vi "RT Loop - Analyze Acceleration_V3.vi"(7 "testing":bool, 8 "error in (no error)":errorcluster, 9 "Acceleration RT FIFO In":T1, 10 "FPGA VI Reference Out 2":refnum<k20>, 11 "Message Queue":refnum<queue>) -> (1 "Acceleration RT FIFO Out":T1)   [LabVIEW 2017]
doc: "Read and analyze acceleration waveform data from FPGA via DMA FIFO. If the acceleration is over the limit, then send the acceleration waveform data to the Log Data Loop."
uses:
  UI Error Handlers/support/Message Queue/Message Cluster.ctl
  controls/Acceleration RT FIFO Reference.ctl
  data_sav.ctl
  Control 1.ctl
  Globals/Global - All RT Loop Stop.vi
  Globals/Global - Configuration Options.vi
  <vilib>/Utility/error.llb/Error Cluster From Error Code.vi
  <vilib>/rvi/errors/niLvFpgaAdjustHostInterfaceError.vi
  <vilib>/rvi/interface/nirviMethod/nirviMethod.xnode
  <vilib>/FPGAPlugInAG/Dynamic/niLvFpga_ReadFifo_Dynamic.vi
  <vilib>/rvi/errors/niLvFpgaMergeErrorWithErrorCode.vi
  UI Error Handlers/support/Logging/Logging.lvlib
  UI Error Handlers/support/Message Queue/Message Queue.lvlib
panel:
  out "error out 2":errorcluster
  out "error out":errorcluster
  out "x-y":u32
  out "G1 status":cluster{"G1 trigger":bool}
  out "G1 status.G1 trigger":bool
  out "sta":bool
  out "logical OR":bool
  in  "Data Rate (Hz)":dbl
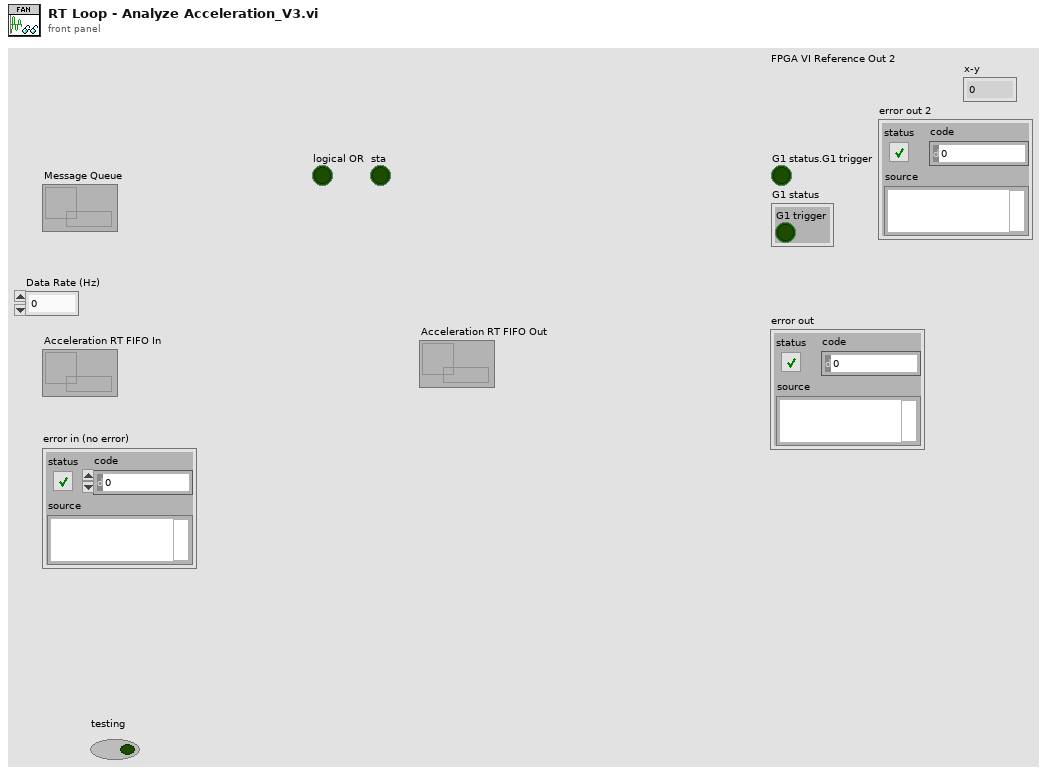
[diagram p1: front panel]
types:
  T1 = typedef "Acceleration RT FIFO Reference.ctl" = refnum<k33>
  T2 = typedef "data_sav.ctl" = cluster{"Log File out 2":refnum<k34>, "Array":T3[]}
  T3 = typedef "Control 1.ctl" = waveform(dbl)
  T4 = cluster{"Tool data":cluster{"Number of teeth":sgl}, "Cutting data":cluster{"rpm":sgl}, "Limits":cluster{"Magnitude threshold":sgl, "Tolerance":sgl}, "G1 status":cluster{"G1 trigger":bool}}
  T5 = cluster{"Log File out":refnum<k34>, waveform(dbl)[]}
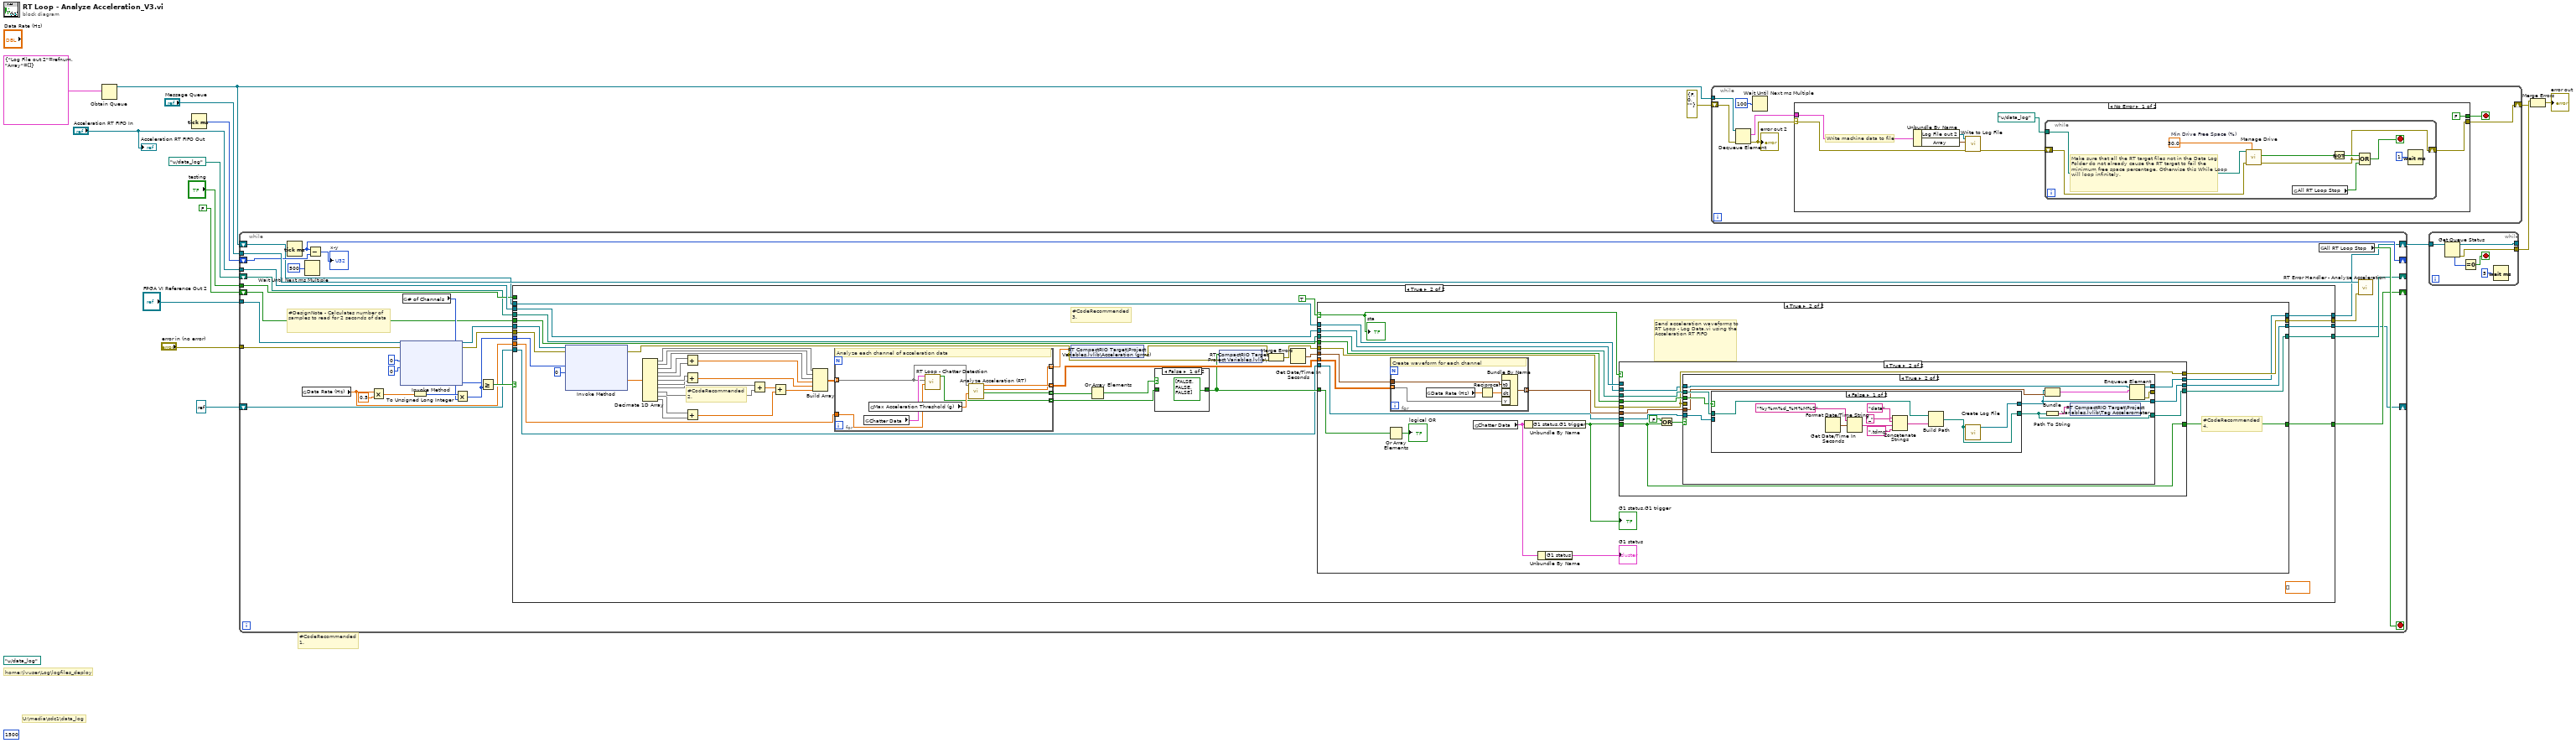
[diagram p0: block diagram]
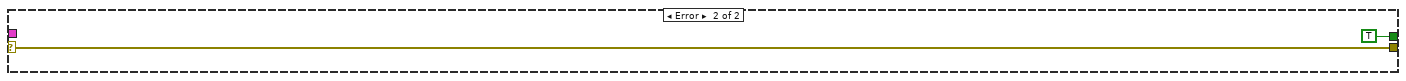
[diagram p2: hidden frame]
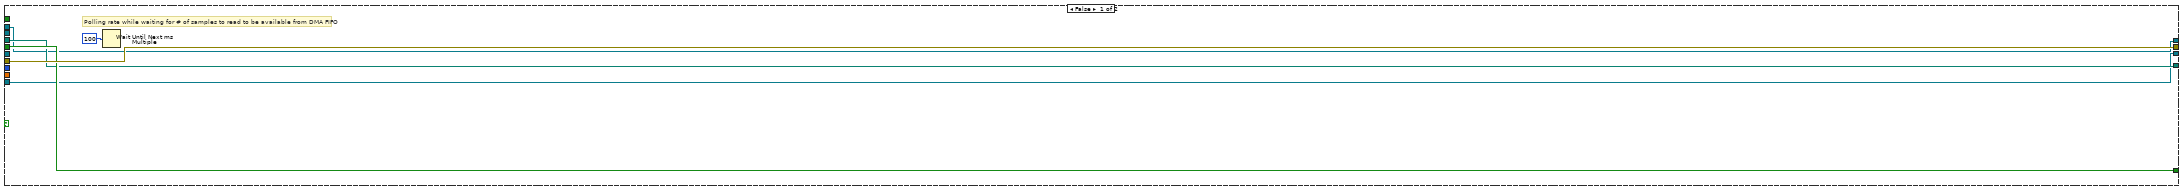
[diagram p3: hidden frame]
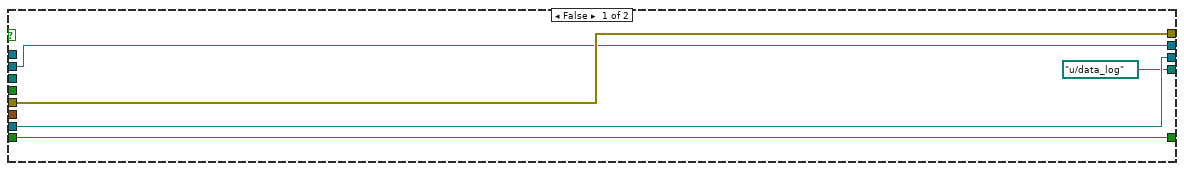
[diagram p6: hidden frame]
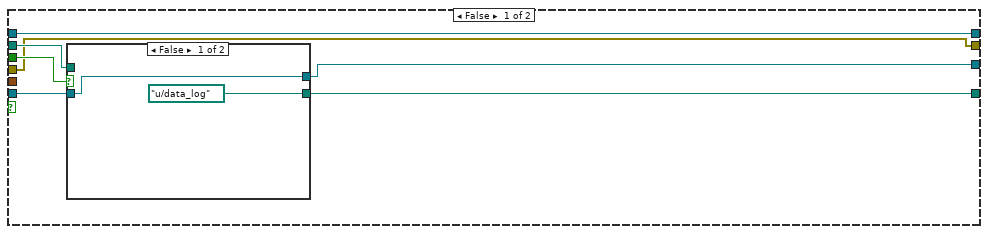
[diagram p7: hidden frame]
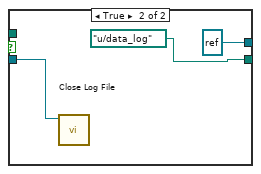
[diagram p8: hidden frame]
diagram:
  (unwired) 1500 ("max queue size (-1, unlimited)")
  (unwired) path "u:/data_log" ("AVI Path")
  # "U:\\media\\sdc1\\data_log"
  # "home:\\lvuser\\Log\\logfiles_deploy"
  # "#CodeRecommended\n1."
  n1 = Obtain Queue(element data type=T2 {"Log File out 2"=refnum, "Array"=[]}) -> (queue out=w5:refnum<queue>)  [unwired: 4 in, 2 out]
  n2 = Tick Count (ms)() -> (millisecond timer value=w9:u32)
  n3 = while {
    tunnel: "FPGA VI Reference Out 2" -> [w47]
    tunnel: "error in (no error)" -> [w46]
    tunnel: "Message Queue" -> [w39]
    tunnel: "Acceleration RT FIFO In" -> [w37]
    tunnel: "testing" -> [w29]
    shift-right: [w26] -> _
    shift-left: path "u:/data_log" ("AVI Path") -> [w25]
    shift-right: [w28] -> _
    shift-left: FALSE -> [w27]
    shift-right: [w24] -> _
    shift-left: refnum<k34> refnum ("Log File out") -> [w23]
    shift-right: [w21] -> _
    shift-left: w9 -> [w22]
    shift-right: [w18] -> w1
    shift-left: w5 -> [w19]
    stop <- w40 stop-if-true
    # "#DesignNote - Calculates number of samples to read for 2 seconds of data"
    n4 = Tick Count (ms)() -> (millisecond timer value=w21:u32)
    n5 = global read "Global - Configuration Options.vi" "Data Rate (Hz)"() -> (w31:dbl)
    n6 = Wait Until Next ms Multiple(millisecond multiple=u32 500) -> ()  [unwired: 1 out]
    n7 = Subtract(x=w21, y=w22) -> (x-y=→"x-y":u32)
    n8 = Multiply(x=w31, y=0.5) -> (x*y=w35:dbl)
    n9 = xnode "Invoke Method"("FPGA VI Reference In"=w47, "error in"=w46, "Number of Elements"=u32 0, "Timeout (ms)"=0) -> ("FPGA VI Reference Out"=w43:refnum<k20>, "error out"=w42:errorcluster, "Elements Remaining"=w30:u32)  [unwired: 1 out]
    n10 = global read "Global - Configuration Options.vi" "# of Channels"() -> (w32:u32)
    n11 = To Unsigned Long Integer(number=w35) -> (unsigned 32bit integer=w34:u32)
    n12 = Multiply(x=w34, y=w32) -> (x*y=w33:u32)
    n13 = Greater Or Equal?(x=w30, y=w33) -> (x >= y?=w41:bool)
    n14 = case shown="True" w41 {
      tunnel: w43 -> [_ w98]
      tunnel: w42 -> [w53 w97]
      tunnel: [w53 w93] -> w38
      tunnel: w33 -> [_ w96]
      tunnel: w37 -> [_ w91]
      tunnel: w31 -> [_ w88]
      tunnel: w29 -> [_ _]
      tunnel: [w51 w80] -> w28
      tunnel: w27 -> [w51 w79]
      tunnel: [w50 w78] -> w26
      tunnel: w25 -> [w50 w77]
      tunnel: [w49 w76] -> w24
      tunnel: w23 -> [w49 w75]
      tunnel: w19 -> [w48 w56]
      tunnel: [w48 w55] -> w18
      frame False {
        # "Polling rate while waiting for # of samples to read to be available from DMA FIFO"
        n15 = Wait Until Next ms Multiple(millisecond multiple=u32 100) -> ()  [unwired: 1 out]
      }
      frame True {
        (unwired) dbl[] []
        # "#CodeRecommended\n3."
        # "#CodeRecommended\n2."
        n16 = xnode "Invoke Method"("FPGA VI Reference In"=w98, "error in"=w97, "Number of Elements"=w96, "Timeout (ms)"=0) -> ("error out"=w87:errorcluster, "Data"=w90:sgl[])  [unwired: 2 out]
        n17 = Decimate 1D Array(w90) -> (w72:sgl[], w71:sgl[], w70:sgl[], w69:sgl[], w68:sgl[], w66:sgl[], w65:sgl[], w64:sgl[], w63:sgl[], w62:sgl[], w61:sgl[])
        n18 = Add(x=w69, y=w68) -> (x+y=w67:sgl[])
        n19 = Add(x=w66, y=w65) -> (x+y=w57:sgl[])
        n20 = Add(x=w62, y=w61) -> (x+y=w59:sgl[])
        n21 = Add(x=w64, y=w63) -> (x+y=w60:sgl[])
        n22 = Add(x=w60, y=w59) -> (x+y=w58:sgl[])
        n23 = Build Array(w72, w71, w70, w67, w57, w58) -> (w73:sgl[][])
        n24 = for {
          tunnel: [w108] -> w92 mode=indexing
          tunnel: [w107] -> w89 mode=indexing
          tunnel: [w106] -> w54 mode=indexing
          tunnel: w88 -> [w104]
          tunnel: [w103] -> w82 mode=indexing
          tunnel: w73 -> [w101] mode=indexing
          # "Analyze each channel of acceleration data"
          n25 = global read "Global - Configuration Options.vi" "Chatter Data"() -> (w102:T4)
          n26 = global read "Global - Configuration Options.vi" "Max Acceleration Threshold (g)"() -> (w105:sgl)
          n27 = call "RT Loop - Chatter Detection.vi"("Data Rate (Hz)"=w104, "Acceleration Waveform (SGL)"=w101, "Chatter Data"=w102) -> ("Chatter?"=w103:bool)  [unwired: 8 in]
          n28 = call "Analyze Acceleration (RT).vi"("Max Instantaneous Acceleration (g)"=w105, "Acceleration Waveform (SGL)"=w101) -> ("Over Limit?"=w108:bool, "Acceleration (grms)"=w106:dbl, "Acceleration Waveform (DBL)"=w107:dbl[])  [unwired: 7 in]
        }
        n29 = shared-variable "RT CompactRIO Target\\Project Variables.lvlib\\Acceleration (grms)"(w54, error in=w87) -> (error out=w85:errorcluster)
        n30 = Or Array Elements(Boolean array=w92) -> (logical OR=w83:bool)
        n31 = case shown="False" w83 {
          tunnel: w82 -> [_ w100]
          tunnel: [bool[] [FALSE, FALSE, FALSE] ("Chatter?") w100] -> w81
          frame False {
          }
          frame True {
          }
        }
        n32 = shared-variable "RT CompactRIO Target\\Project Variables.lvlib\\Chatter?"(w81, error in=w87) -> (error out=w86:errorcluster)
        n33 = Merge Errors(w85, w86) -> (w84:errorcluster)
        n34 = Get Date/Time In Seconds() -> (seconds since 1Jan1904=w94:timestamp)
        n35 = case shown="True" TRUE {
          selector: TRUE -> [_ w114]
          tunnel: w94 -> [_ w133]
          tunnel: w84 -> [w113 w132]
          tunnel: [w113 w117] -> w93
          tunnel: w91 -> [_ w130]
          tunnel: w89 -> [_ w129]
          tunnel: w81 -> [_ w127]
          tunnel: [w112 w124] -> w80
          tunnel: w79 -> [w112 w123]
          tunnel: [w111 w122] -> w78
          tunnel: w77 -> [w111 w118]
          tunnel: [w110 w121] -> w76
          tunnel: w75 -> [w110 w120]
          tunnel: w56 -> [w109 w116]
          tunnel: [w109 w115] -> w55
          frame False {
          }
          frame True {
            # "#CodeRecommended\n4."
            # "Send acceleration waveforms to RT Loop - Log Data.vi using the Acceleration RT FIFO"
            n36 = Or Array Elements(Boolean array=w127) -> (logical OR=→"logical OR":bool)
            n37 = for {
              tunnel: w129 -> [w190] mode=indexing
              tunnel: w133 -> [w189]
              tunnel: [w187] -> w131 mode=indexing
              # "Create waveform for each channel"
              n38 = global read "Global - Configuration Options.vi" "Data Rate (Hz)"() -> (w186:dbl)
              n39 = Reciprocal(x=w186) -> (1/x=w188:dbl)
              n40 = Bundle By Name("t0"=w189, "dt"=w188, "Y"=w190) -> (w187:waveform(dbl))  [unwired: 1 in]
            }
            n41 = global read "Global - Configuration Options.vi" "Chatter Data"() -> (w126:T4)
            n42 = Unbundle By Name(w126) -> ("G1 status.G1 trigger"=w119:bool)
            "G1 status.G1 trigger" <- w119
            n43 = Unbundle By Name(w126) -> ("G1 status"=→"G1 status":cluster{"G1 trigger":bool})
            n44 = case shown="True" w114 {
              tunnel: w132 -> [w138 w141]
              tunnel: w131 -> [_ w142]
              tunnel: w130 -> [_ _]
              tunnel: w119 -> [w136 w148]
              tunnel: [w136 w148] -> w124
              tunnel: w123 -> [_ w147]
              tunnel: [path "u:/data_log" ("AVI Path") w146] -> w122
              tunnel: w118 -> [_ w145]
              tunnel: [w137 w144] -> w121
              tunnel: w120 -> [w137 w143]
              tunnel: [w138 w141] -> w117
              tunnel: w116 -> [w134 w139]
              tunnel: [w134 w140] -> w115
              frame False {
              }
              frame True {
                n45 = Or(x=FALSE, y=w148) -> (x .or. y?=w150:bool)
                n46 = case shown="True" w150 {
                  tunnel: w145 -> [w154 w173]
                  tunnel: [w157 w170] -> w146
                  tunnel: w147 -> [w155 w172]
                  tunnel: w143 -> [w156 w164]
                  tunnel: w142 -> [_ w166]
                  tunnel: [w153 w163] -> w144
                  tunnel: w141 -> [w152 _]
                  tunnel: [w152 w169] -> _
                  tunnel: w139 -> [w151 w165]
                  tunnel: [w151 w168] -> w140
                  frame False {
                    n47 = case shown="False" w155 {
                      tunnel: [path "u:/data_log" ("AVI Path") path "u:/data_log" ("AVI Path")] -> w157
                      tunnel: w156 -> [w158 w161]
                      tunnel: w154 -> [_ _]
                      tunnel: [w158 refnum<k34> refnum ("Log File out")] -> w153
                      frame False {
                      }
                      frame True {
                        n48 = call "Close Log File.vi"("tdms file"=w161) -> ()  [unwired: 10 in, 1 out]
                      }
                    }
                  }
                  frame True {
                    n49 = case shown="False" w172 {
                      tunnel: w173 -> [w176 w185]
                      tunnel: [w175 w185] -> w170
                      tunnel: [w174 w184] -> w163
                      tunnel: w164 -> [_ w184]
                      frame False {
                        n50 = Get Date/Time In Seconds() -> (seconds since 1Jan1904=w179:timestamp)
                        n51 = Format Date/Time String(time format string (%c)="%y%m%d_%H%M%S", seconds (now)=w179) -> (date/time string=w182:string)  [unwired: 1 out]
                        n52 = Concatenate Strings("data" ("string"), "_" ("string"), w182, ".tdms" ("string")) -> (w177:string)
                        n53 = Build Path(base path=w176, name or relative path=w177) -> (appended path=w175:path)
                        n54 = call "Create Log File.vi"("Acceleration Exceeded Log Folder"=w175) -> ("Log File out"=w174:refnum<k34>)  [unwired: 9 in, 1 out]
                      }
                      frame True {
                      }
                    }
                    n55 = Path To String(path=w170) -> (string=w171:string)
                    n56 = Bundle("Log File out"=w163, w166) -> (w167:T5)  [unwired: 1 in]
                    n57 = shared-variable "RT CompactRIO Target\\Project Variables.lvlib\\Tag Accelerometer"(w171) -> ()  [unwired: 1 in, 1 out]
                    n58 = Enqueue Element(queue=w165, element=w167) -> (queue out=w168:refnum<queue>, error out=w169:errorcluster)  [unwired: 2 in, 1 out]
                  }
                }
              }
            }
            "sta" <- w114
          }
        }
      }
    }
    n59 = global read "Global - All RT Loop Stop.vi" "All RT Loop Stop"() -> (w40:bool)
    n60 = call "RT Error Handler - Analyze Acceleration.vi"("error in (no error)"=w38, "Message Queue"=w39) -> ()  [unwired: 9 in, 1 out]
  }
  n61 = while {
    tunnel: w5 -> [w192]
    shift-right: [w194] -> w4
    shift-left: errorcluster {"status"=FALSE, "code"=0, "source"=""} ("error IO") -> [w197]
    stop <- w195 stop-if-true
    n62 = Dequeue Element(queue=w192, error in (no error)=w197) -> (element=w193:T2, error out=w196:errorcluster)  [unwired: 1 in, 2 out]
    "error out 2" <- w196
    n63 = Wait Until Next ms Multiple(millisecond multiple=u32 100) -> ()  [unwired: 1 out]
    n64 = case shown="No Error" w196 {
      selector: w196 -> [w201 w215]
      tunnel: [FALSE TRUE] -> w195
      tunnel: [w203 w215] -> w194
      tunnel: w193 -> [w200 _]
      frame No Error {
        # "Write machine data to file"
        n65 = Unbundle By Name(w200) -> ("Log File out 2"=w199:refnum<k34>, "Array"=w198:T3[])
        n66 = call "Write to Log File.vi"("error in (no error)"=w201, "Array of Waveforms"=w198, "Log File in"=w199) -> ("error out"=w202:errorcluster)  [unwired: 7 in, 1 out]
        n67 = while {
          shift-right: [w209] -> w203
          shift-left: w202 -> [w210]
          tunnel: path "u:/data_log" ("AVI Path") -> [w207]
          stop <- w214 stop-if-true
          w208 = 30.0  # Min Drive Free Space (%)
          # "Make sure that all the RT target files not in the Data Log Folder do not already cause the RT target to fail the minimum free space percentage. Otherwise this While Loop will loop infinitely."
          n68 = call "Manage Drive.vi"("Min Drive Free Space (%)"=w208, "error in"=w210, "Data Folder"=w207) -> ("error out"=w209:errorcluster, "Drive Space Below Limit"=w206:bool)  [unwired: 7 in]
          n69 = global read "Global - All RT Loop Stop.vi" "All RT Loop Stop"() -> (w211:bool)
          n70 = Not(x=w206) -> (.not. x?=w213:bool)
          n71 = Compound Arithmetic op=OR(w213, w209, w211) -> (w214:bool)
          n72 = Wait (ms)(milliseconds to wait=u32 1) -> ()  [unwired: 1 out]
        }
      }
      frame Error {
      }
    }
  }
  n73 = while {
    tunnel: [w221] -> w7
    tunnel: [w219] -> _
    tunnel: w1 -> [w217]
    stop <- w220 stop-if-true
    n74 = Get Queue Status(queue=w217) -> (queue out=w219:refnum<queue>, error out=w221:errorcluster, # elements in queue=w218:i32)  [unwired: 2 in, 5 out]
    n75 = Equal To 0?(x=w218) -> (x = 0?=w220:bool)
    n76 = Wait (ms)(milliseconds to wait=u32 5) -> ()  [unwired: 1 out]
  }
  n77 = Merge Errors(w7, w4) -> (→"error out":errorcluster)
  "Acceleration RT FIFO Out" <- "Acceleration RT FIFO In"
